vi "Write User ID.vi"(8 "Error In":errorcluster, 10 "User ID":u32, 11 "SFTP Attributes In":refnum<class "SFTP Attributes.lvclass">) -> (0 "Error Out":errorcluster, 3 "SFTP Attribute Out":refnum<class "SFTP Attributes.lvclass">)   [LabVIEW 2018, in "Toolkit.lvlib" / "SFTP Attributes.lvclass"]
uses:
  SFTP Attributes.lvclass
  SFTP Attributes.lvclass/SFTP Attributes.ctl
  SSH/SSH.lvclass/SSH.ctl
  Toolkit.lvlib
  SSH/SSH.lvclass
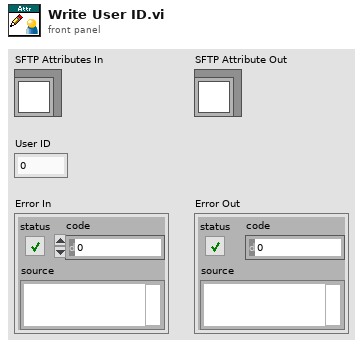
[diagram p1: front panel]
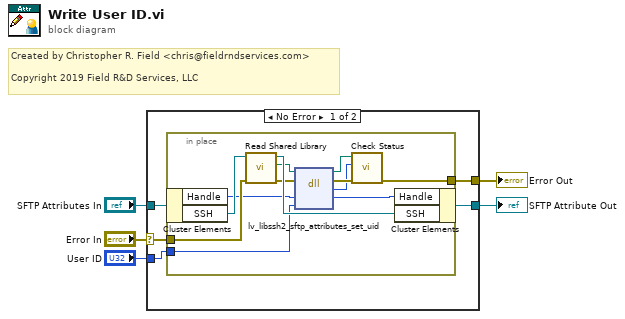
[diagram p0: block diagram]
diagram:
  # "Created by Christopher R. Field <chris@fieldrndservices.com>\n\nCopyright 2019 Field R&D Services, LLC"
  n1 = case shown="No Error" "Error In" {
    selector: "Error In" -> [w9 w24]
    tunnel: [w7 w24] -> w4
    tunnel: "SFTP Attributes In" -> [w10 w23]
    tunnel: [w8 w23] -> w2
    tunnel: "User ID" -> [w6 _]
    frame No Error {
      n2 = in-place {
        in-place-border: w9 -> [w15]
        in-place-border: [w12] -> w7
        in-place-border: w6 -> [w11]
        n3 = in-place-cluster #1(w10) -> ("Handle"=w14:u64, "SSH"=w19:refnum<class "SSH.lvclass">)
        n4 = call "Read Shared Library.vi"("Error In"=w15, "SSH In"=w19) -> ("Error Out"=w16:errorcluster, "lv-libssh2 Shared Library"=w17:path, "SSH Out"=w18:refnum<class "SSH.lvclass">)  [unwired: 7 in]
        n5 = dll-call lib="lv-libssh2.*" fn="lv_libssh2_sftp_attributes_set_uid"(path in=w17, error in=w16, "handle"=w14, "uid"=w11) -> (path out=w21:path, error out=w22:errorcluster, "status"=w20:i32, "handle"=w13:u64)  [unwired: 2 in]
        n6 = call "Check Status.vi"("Error In"=w22, "Status"=w20, "lv-libssh2 Shared Library In"=w21) -> ("Error Out"=w12:errorcluster)  [unwired: 7 in, 1 out]
        n7 = in-place-cluster #1("Handle"=w13, "SSH"=w18) -> (w8:refnum<class "SFTP Attributes.lvclass">)
      }
    }
    frame Error {
    }
  }
  "Error Out" <- w4
  "SFTP Attribute Out" <- w2
